vi "boolean cluster to enum.vi"(11 "Valid User Options":T2) -> (3 "User Options":T1=enum."Create account")   [LabVIEW 2015, in "AguaClara Library.lvlib"]
uses:
  AguaClara Library.lvlib
  Register options.ctl
  User status cmd.ctl
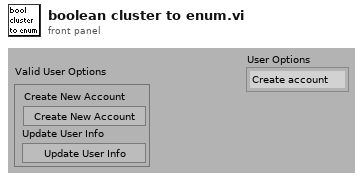
[diagram p1: front panel]
types:
  T1 = typedef "AguaClara Library.lvlib/User status cmd.ctl" = enum16{"Load File Path", "Create account", "Update user", "Email password", "Load inputs", "Check status"}
  T2 = typedef "AguaClara Library.lvlib/Register options.ctl" = cluster{"New Account":bool, "Update User Info":bool}
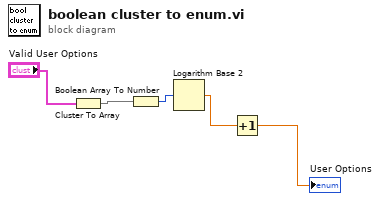
[diagram p0: block diagram]
diagram:
  n1 = Cluster To Array(cluster="Valid User Options") -> (array=w4:bool[])
  n2 = Boolean Array To Number(Boolean array=w4) -> (number=w3:u32)
  n3 = Logarithm Base 2(1:w3) -> (0:w2:dbl)
  n4 = Increment(x=w2) -> (x+1=→"User Options":dbl)
